vi "marshalling.vi"(8 "error in (no error)":errorcluster, 10 "Variant":variant, 11 "Serializer":refnum<class "Serializer.easyXML.lvclass">) -> (0 "error out":errorcluster, 2 "XML String":string, 3 "Serializer out":refnum<class "Serializer.easyXML.lvclass">)   [LabVIEW 2019, in "OpenSerializer.easyXML.lvlib" / "Serializer.easyXML.lvclass"]
uses:
  Serializer.easyXML.lvclass
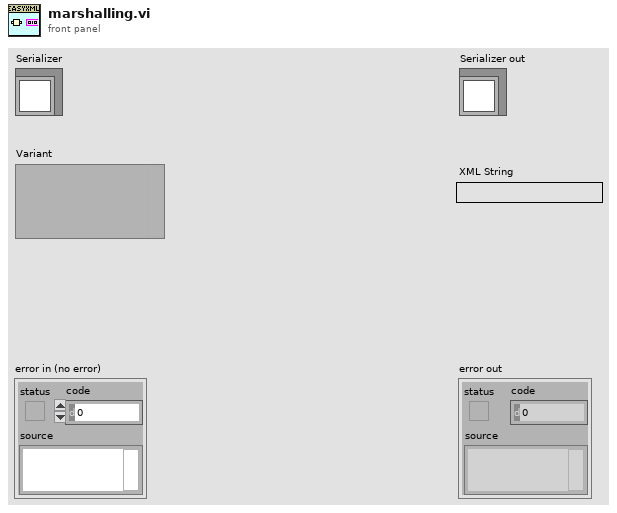
[diagram p1: front panel]
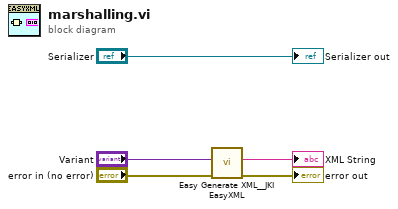
[diagram p0: block diagram]
diagram:
  n1 = call <vilib>:"Easy Generate XML__JKI EasyXML.vi"("error in (no error)"="error in (no error)", "LabVIEW Data"="Variant") -> ("error out"=→"error out":errorcluster, "XML String"=→"XML String":string)  [unwired: 8 in]
  "Serializer out" <- "Serializer"
